vi "calculate_rms_coef.vi"(9 "Array 2":waveform(dbl)[](array[waveform]), 10 "DC":dbl[](array[numeric]), 11 "measured_value":dbl[](array[numeric])) -> (2 "coef_values":dbl[](array[numeric]), 3 "RMS values":dbl[](array[numeric]) format="%.2p")   [LabVIEW 2017]
uses:
  <vilib>/measure/madcrms.llb/Basic Averaged DC-RMS for N Chan.vi
  <vilib>/measure/NI_MAPro.lvlib
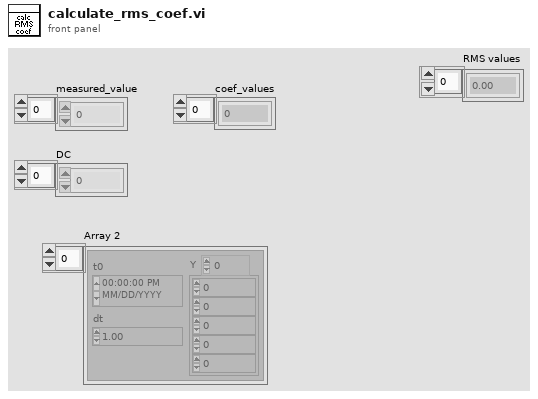
[diagram p1: front panel]
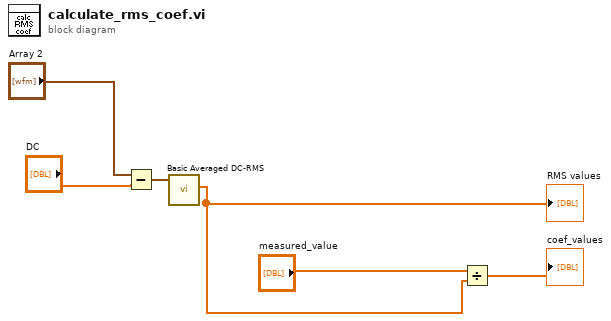
[diagram p0: block diagram]
diagram:
  n1 = Subtract(x="Array 2", y="DC") -> (x-y=w4:waveform(dbl)[])
  n2 = call-poly <vilib>:"Basic Averaged DC-RMS.vi"("signals in"=w4) -> ("RMS values"=w1:dbl[])  [unwired: 7 in, 3 out]
  "RMS values" <- w1
  n3 = Divide(x="measured_value", y=w1) -> (x/y=→"coef_values":dbl[])
